vi "Punto 3 _ JUAN BERMUDEZ.vi"() -> ()   [LabVIEW 2020]
panel:
  out "Array 3":dbl[](array[numeric])
  in  "Array 5":dbl[](array[numeric])
  out "Array 2":dbl[](array[numeric])
  in  "Array 4":dbl[](array[numeric])
  in  "Array 3":dbl[](array[numeric])
  out "Array 1":dbl[](array[numeric])
  in  "Array":dbl[](array[numeric])
  # "Juan Bermudez"
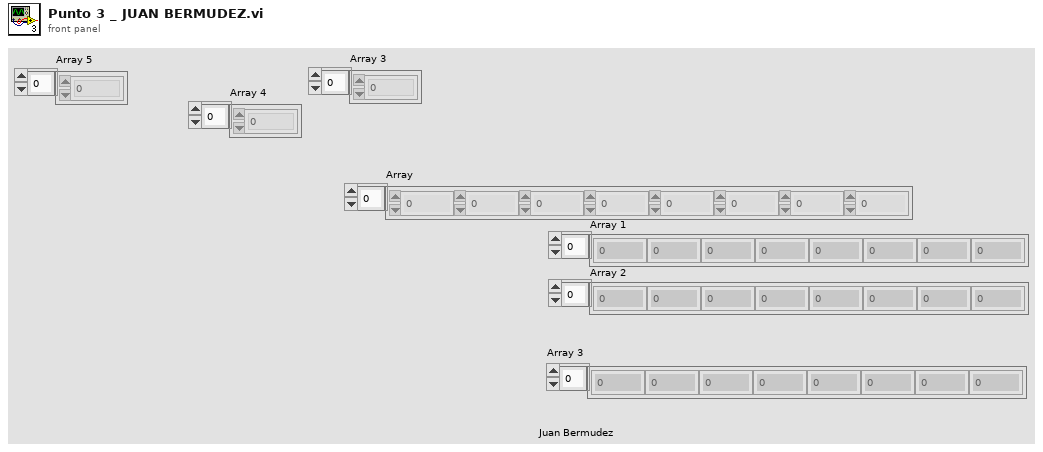
[diagram p1: front panel]
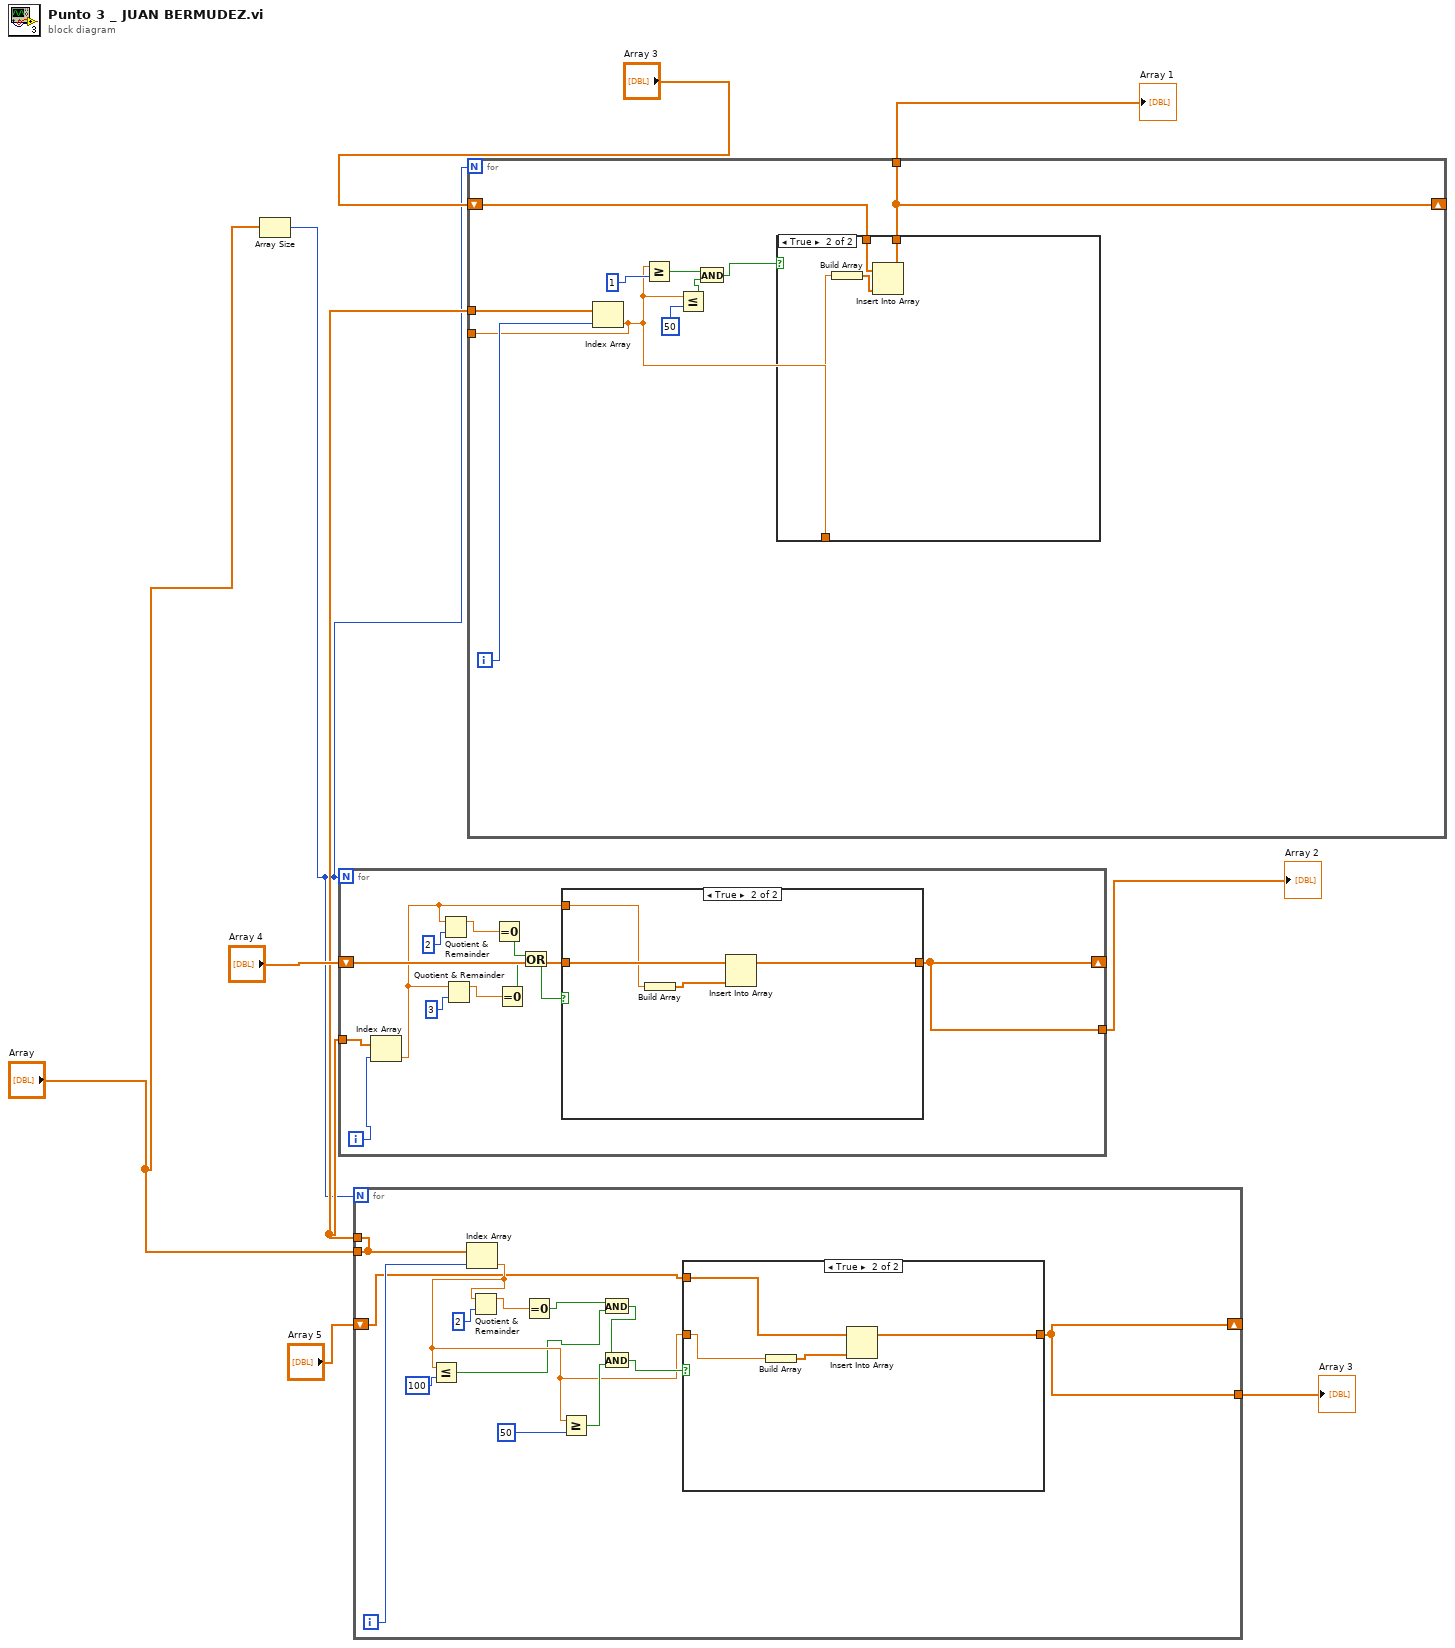
[diagram p0: block diagram]
diagram:
  n1 = Array Size(array="Array") -> (size(s)=w1:i32)
  n2 = for {
    N: w1 -> [_]
    tunnel: "Array" -> [w16]
    tunnel: [w16] -> w5
    shift-right: [w13] -> _
    shift-left: "Array 5" -> [w14]
    tunnel: [w13] -> w3
    i -> [w21]
    n3 = Index Array(array=w16, index=w21) -> (element=w15:dbl)
    n4 = Less Or Equal?(x=w15, y=100) -> (x <= y?=w11:bool)
    n5 = Quotient & Remainder(x=w15, y=2) -> (x-y*floor(x/y)=w22:dbl)  [unwired: 1 out]
    n6 = Equal To 0?(x=w22) -> (x = 0?=w12:bool)
    n7 = Greater Or Equal?(x=w15, y=50) -> (x >= y?=w18:bool)
    n8 = And(x=w12, y=w11) -> (x .and. y?=w10:bool)
    n9 = And(x=w10, y=w18) -> (x .and. y?=w17:bool)
    n10 = case shown="True" w17 {
      tunnel: w15 -> [_ w28]
      tunnel: [w24 w25] -> w13
      tunnel: w14 -> [w24 w26]
      frame False {
      }
      frame True {
        n11 = Build Array(w28) -> (w27:dbl[])
        n12 = Insert Into Array(array=w26, new element=w27) -> (w25:dbl[])  [unwired: 1 in]
      }
    }
  }
  "Array 3" <- w3
  n13 = for {
    N: w1 -> [_]
    shift-right: [w39] -> _
    shift-left: "Array 4" -> [w40]
    tunnel: [w39] -> w6
    tunnel: w5 -> [w31]
    i -> [w29]
    n14 = Index Array(array=w31, index=w29) -> (element=w30:dbl)
    n15 = Quotient & Remainder(x=w30, y=2) -> (x-y*floor(x/y)=w35:dbl)  [unwired: 1 out]
    n16 = Quotient & Remainder(x=w30, y=3) -> (x-y*floor(x/y)=w36:dbl)  [unwired: 1 out]
    n17 = Equal To 0?(x=w35) -> (x = 0?=w37:bool)
    n18 = Equal To 0?(x=w36) -> (x = 0?=w38:bool)
    n19 = Or(x=w37, y=w38) -> (x .or. y?=w32:bool)
    n20 = case shown="True" w32 {
      tunnel: w40 -> [w41 w44]
      tunnel: [w41 w43] -> w39
      tunnel: w30 -> [_ w42]
      frame False {
      }
      frame True {
        n21 = Build Array(w42) -> (w45:dbl[])
        n22 = Insert Into Array(array=w44, new element=w45) -> (w43:dbl[])  [unwired: 1 in]
      }
    }
  }
  "Array 2" <- w6
  n23 = for {
    N: w1 -> [_]
    tunnel: w5 -> [w53]
    shift-right: [w47] -> _
    shift-left: "Array 3" -> [w48]
    tunnel: [w47] -> w8
    tunnel: [w46] -> _
    i -> [w54]
    n24 = Index Array(array=w53, index=w54) -> (element=w46:dbl)
    n25 = Greater Or Equal?(x=w46, y=1) -> (x >= y?=w51:bool)
    n26 = Less Or Equal?(x=w46, y=50) -> (x <= y?=w50:bool)
    n27 = And(x=w51, y=w50) -> (x .and. y?=w49:bool)
    n28 = case shown="True" w49 {
      tunnel: w46 -> [_ w60]
      tunnel: w48 -> [w56 w58]
      tunnel: [w56 w57] -> w47
      frame False {
      }
      frame True {
        n29 = Build Array(w60) -> (w59:dbl[])
        n30 = Insert Into Array(array=w58, new element=w59) -> (w57:dbl[])  [unwired: 1 in]
      }
    }
  }
  "Array 1" <- w8
